vi "Close VacuumPlus (subVi).vi"(2 "error in (no error)":errorcluster) -> (0 "error out":errorcluster, 1 "standard output":string)   [LabVIEW 2016]
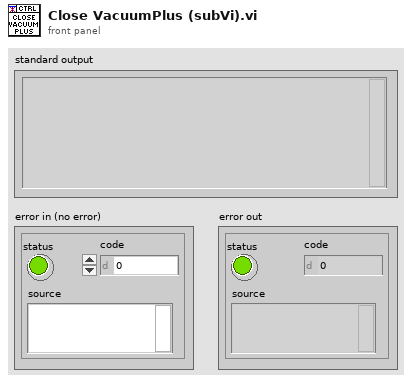
[diagram p1: front panel]
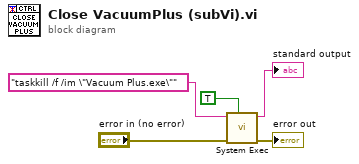
[diagram p0: block diagram]
diagram:
  n1 = call <vilib>:"System Exec.vi"("wait until completion? (T)"=TRUE, "error in (no error)"="error in (no error)", "command line"="taskkill /f /im \"Vacuum Plus.exe\"") -> ("error out"=→"error out":errorcluster, "standard output"=→"standard output":string)  [unwired: 5 in, 2 out]
